vi "(SubVI)Waveform Editor_Import Manager.vi"(5 "New?":bool, 7 "Sampling Rate In":dbl, 8 "error in (no error)":errorcluster caption="에러 입력(에러 없음)", 10 "File Path":path, 11 "WAV File.lvclass":refnum<class "WAV File.lvclass">) -> (0 "error out":errorcluster caption="에러 출력", 2 "Apply?":bool, 3 "*.WAV Data":refnum<class "WAV File.lvclass">)   [LabVIEW 2020]
uses:
  Libraries/Waveform Obj Class/WAV File/WAV File.lvclass
  <vilib>/Utility/miscctls.llb/LVPointTypeDef.ctl
  Libraries/Waveform Obj Class/WAV File/WAV File.lvclass/WAV File.ctl
  Libraries/Waveform Obj Class/Waveform File/Waveform File.lvclass/Waveform File.ctl
  Libraries/Waveform Obj Class/Waveform Obj/Waveform Obj.lvclass/Waveform Obj.ctl
  Libraries/Waveform Obj Class/WAV File/Accessors/Read sound format.vi
  Libraries/Waveform Obj Class/Waveform File/Accessors/Read channel.vi
  Libraries/Waveform Obj Class/Waveform Obj/Accessors/Read voltage range.vi
  Libraries/Waveform Obj Class/Waveform Obj/Accessors/Read wait.vi
  Libraries/Waveform Obj Class/Waveform Obj/Accessors/Write sampling rate.vi
  Libraries/Waveform Obj Class/Waveform File/Accessors/Write channel.vi
  Libraries/Waveform Obj Class/WAV File/Accessors/Write normalize.vi
  Libraries/Waveform Obj Class/Waveform Obj/Accessors/Write wait.vi
  Libraries/Waveform Obj Class/Waveform Obj/Accessors/Write voltage range.vi
  Variables/(Var)System Variables.vi
  Libraries/Haptic IC Class/Haptic IC/Haptic IC.lvclass
panel:
  in  "Wait":u8(ring) items=["0us", "166us", "332us", "498us", "664us", "830us", "996us", "1162us", "1328us", "1494us", "1660us", "1826us", "1992us", "2158us", "2324us", "2490us"]
  in  "Normalize":bool=TRUE
  out "Bits per Sample":i32 caption="Bits / Sample"
  in  "Apply":bool
  out "Sampling Rate":dbl format="%#pHz"
  out "Graph":waveform(dbl)[](graph)
  in  "Voltage Range":dbl(ring) caption="VD Clamp" items=["0.00V"=0.0, "0.04V"=0.04, "0.08V"=0.08, "0.12V"=0.12, "0.16V"=0.16, "0.20V"=0.2, "0.24V"=0.24, "0.28V"=0.28, "0.32V"=0.32, "0.36V"=0.36, "0.40V"=0.4, "0.44V"=0.44, "0.48V"=0.48, "0.52V"=0.52, "0.56V"=0.56, "0.60V"=0.6, "0.64V"=0.64, "0.68V"=0.68, "0.72V"=0.72, "0.76V"=0.76, "0.80V"=0.8, "0.84V"=0.84, "0.88V"=0.88, "0.92V"=0.92, "0.96V"=0.96, "1.00V"=1.0, "1.04V"=1.04, "1.08V"=1.08, "1.12V"=1.12, "1.16V"=1.16, "1.20V"=1.2, "1.24V"=1.24, "1.28V"=1.28, "1.32V"=1.32, "1.36V"=1.36, "1.40V"=1.4, "1.44V"=1.44, "1.48V"=1.48, "1.52V"=1.52, "1.56V"=1.56, "1.60V"=1.6, "1.64V"=1.64, "1.68V"=1.68, "1.72V"=1.72, "1.76V"=1.76, "1.80V"=1.8, "1.84V"=1.84, "1.88V"=1.88, "1.92V"=1.92, "1.96V"=1.96, "2.00V"=2.0, "2.04V"=2.04, "2.08V"=2.08, "2.12V"=2.12, "2.16V"=2.16, "2.20V"=2.2, "2.24V"=2.24, "2.28V"=2.28, "2.32V"=2.32, "2.36V"=2.36, "2.40V"=2.4, "2.44V"=2.44, "2.48V"=2.48, "2.52V"=2.52, "2.56V"=2.56, "2.60V"=2.6, "2.64V"=2.64, "2.68V"=2.68, "2.72V"=2.72, "2.76V"=2.76, "2.80V"=2.8, "2.84V"=2.84, "2.88V"=2.88, "2.92V"=2.92, "2.96V"=2.96, "3.00V"=3.0, "3.04V"=3.04, "3.08V"=3.08, "3.12V"=3.12, "3.16V"=3.16, "3.20V"=3.2, "3.24V"=3.24, "3.28V"=3.28, "3.32V"=3.32, "3.36V"=3.36, "3.40V"=3.4, "3.44V"=3.44, "3.48V"=3.48, "3.52V"=3.52, "3.56V"=3.56, "3.60V"=3.6, "3.64V"=3.64, "3.68V"=3.68, "3.72V"=3.72, "3.76V"=3.76, "3.80V"=3.8, "3.84V"=3.84, "3.88V"=3.88, "3.92V"=3.92, "3.96V"=3.96, "4.00V"=4.0, "4.04V"=4.04, "4.08V"=4.08, "4.12V"=4.12, "4.16V"=4.16, "4.20V"=4.2, "4.24V"=4.24, "4.28V"=4.28, "4.32V"=4.32, "4.36V"=4.36, "4.40V"=4.4, "4.44V"=4.44, "4.48V"=4.48, "4.52V"=4.52, "4.56V"=4.56, "4.60V"=4.6, "4.64V"=4.64, "4.68V"=4.68, "4.72V"=4.72, "4.76V"=4.76, "4.80V"=4.8, "4.84V"=4.84, "4.88V"=4.88, "4.92V"=4.92, "4.96V"=4.96, "5.00V"=5.0, "5.04V"=5.04, "5.08V"=5.08, "5.12V"=5.12, "5.16V"=5.16, "5.20V"=5.2, "5.24V"=5.24, "5.28V"=5.28, "5.32V"=5.32, "5.36V"=5.36, "5.40V"=5.4, "5.44V"=5.44, "5.48V"=5.48, "5.52V"=5.52, "5.56V"=5.56, "5.60V"=5.6, "5.64V"=5.64, "5.68V"=5.68, "5.72V"=5.72, "5.76V"=5.76, "5.80V"=5.8, "5.84V"=5.84, "5.88V"=5.88, "5.92V"=5.92, "5.96V"=5.96, "6.00V"=6.0, "6.04V"=6.04, "6.08V"=6.08, "6.12V"=6.12, "6.16V"=6.16, "6.20V"=6.2, "6.24V"=6.24, "6.28V"=6.28, "6.32V"=6.32, "6.36V"=6.36, "6.40V"=6.4, "6.44V"=6.44, "6.48V"=6.48, "6.52V"=6.52, "6.56V"=6.56, "6.60V"=6.6, "6.64V"=6.64, "6.68V"=6.68, "6.72V"=6.72, "6.76V"=6.76, "6.80V"=6.8, "6.84V"=6.84, "6.88V"=6.88, "6.92V"=6.92, "6.96V"=6.96, "7.00V"=7.0, "7.04V"=7.04, "7.08V"=7.08, "7.12V"=7.12, "7.16V"=7.16, "7.20V"=7.2, "7.24V"=7.24, "7.28V"=7.28, "7.32V"=7.32, "7.36V"=7.36, "7.40V"=7.4, "7.44V"=7.44, "7.48V"=7.48, "7.52V"=7.52, "7.56V"=7.56, "7.60V"=7.6, "7.64V"=7.64, "7.68V"=7.68, "7.72V"=7.72, "7.76V"=7.76, "7.80V"=7.8, "7.84V"=7.84, "7.88V"=7.88, "7.92V"=7.92, "7.96V"=7.96, "8.00V"=8.0, "8.04V"=8.04, "8.08V"=8.08, "8.12V"=8.12, "8.16V"=8.16, "8.20V"=8.2, "8.24V"=8.24, "8.28V"=8.28, "8.32V"=8.32, "8.36V"=8.36, "8.40V"=8.4, "8.44V"=8.44, "8.48V"=8.48, "8.52V"=8.52, "8.56V"=8.56, "8.60V"=8.6, "8.64V"=8.64, "8.68V"=8.68, "8.72V"=8.72, "8.76V"=8.76, "8.80V"=8.8, "8.84V"=8.84, "8.88V"=8.88, "8.92V"=8.92, "8.96V"=8.96, "9.00V"=9.0, "9.04V"=9.04, "9.08V"=9.08, "9.12V"=9.12, "9.16V"=9.16, "9.20V"=9.2, "9.24V"=9.24, "9.28V"=9.28, "9.32V"=9.32, "9.36V"=9.36, "9.40V"=9.4, "9.44V"=9.44, "9.48V"=9.48, "9.52V"=9.52, "9.56V"=9.56, "9.60V"=9.6, "9.64V"=9.64, "9.68V"=9.68, "9.72V"=9.72, "9.76V"=9.76, "9.80V"=9.8, "9.84V"=9.84, "9.88V"=9.88, "9.92V"=9.92, "9.96V"=9.96, "10.00V"=10.0, "10.04V"=10.04, "10.08V"=10.08, "10.12V"=10.12, "10.16V"=10.16, "10.20V"=10.2]
  out "Freq":dbl caption="Sampling Rate" format="%#pHz"
  in  "Channel":i32(ring) items=["0"]
  # "Import Manager"
  # "File Info"
  # "Resampling"
  # "Setting"
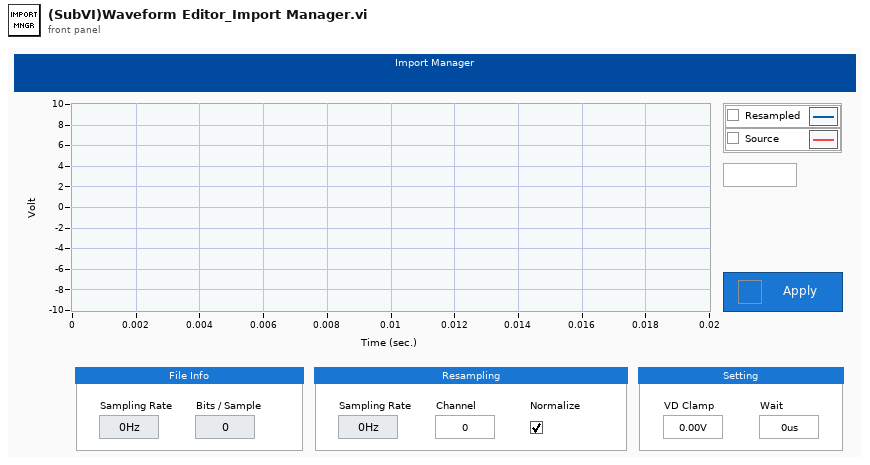
[diagram p1: front panel]
types:
  T1 = typedef "LVPointTypeDef.ctl" = cluster{"Horizontal":i16, "Vertical":i16}
  T2 = typedef "LVStringsAndValuesArrayTypeDef_DBL.ctl" = cluster{"String":string, "Value":dbl}[]
  T3 = typedef "LVStringsAndValuesArrayTypeDef_U8.ctl" = cluster{"String":string, "Value":u8}[]
  T4 = typedef "Sound Data Format.ctl" = cluster{"sample rate (S/s)":dbl, "number of channels":i32, "bits per sample":i32}
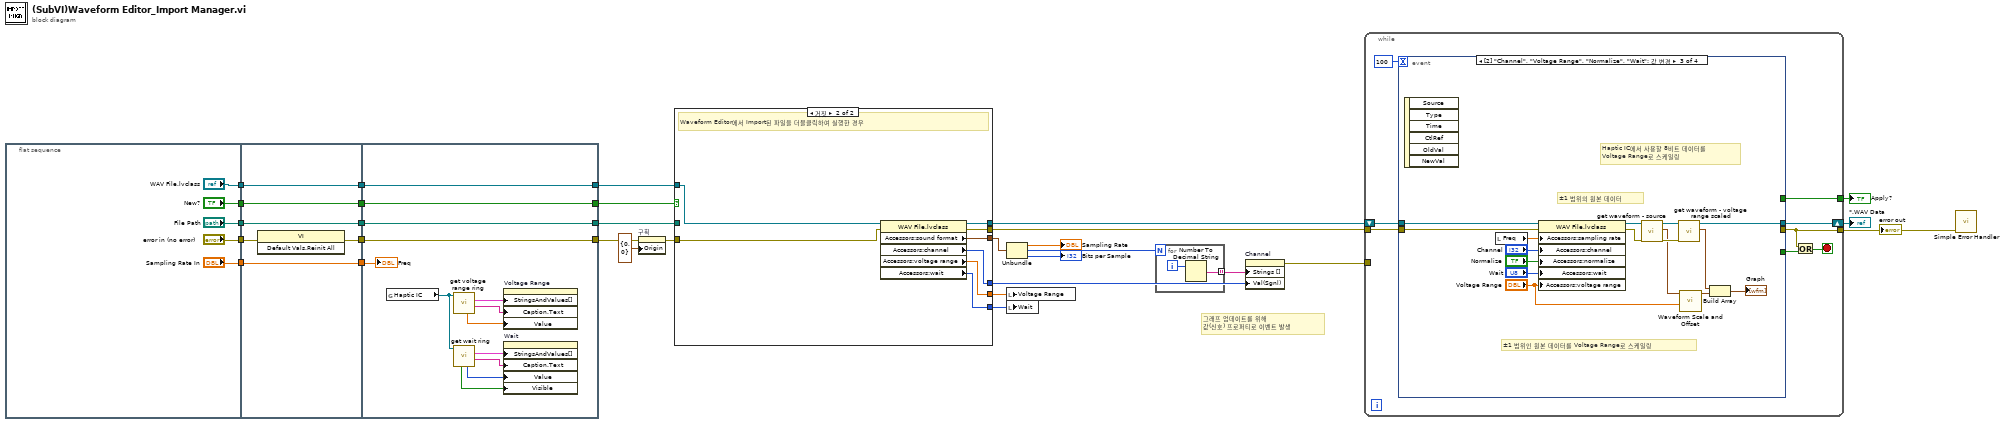
[diagram p0: block diagram]
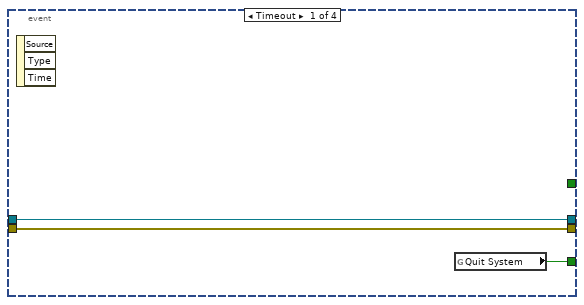
[diagram p2: hidden frame]
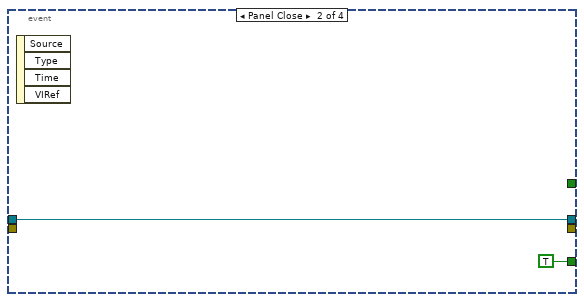
[diagram p3: hidden frame]
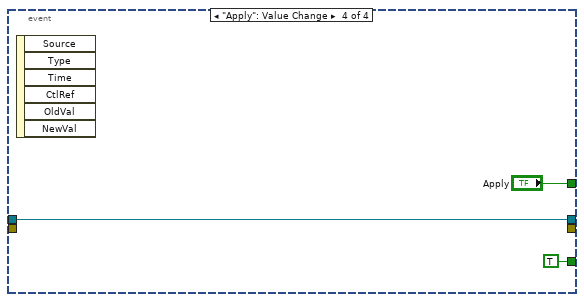
[diagram p4: hidden frame]
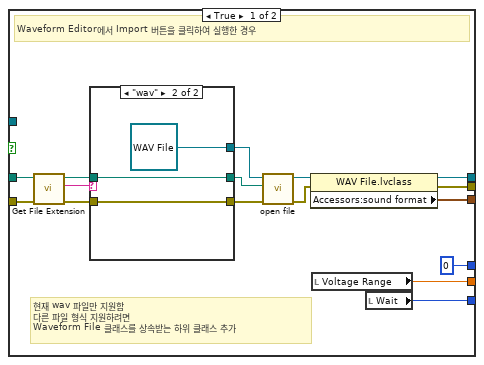
[diagram p5: hidden frame]
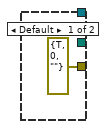
[diagram p6: hidden frame]
diagram:
  # "그래프 업데이트를 위해\n값(신호) 프로퍼티로 이벤트 발생"
  n1 = flat-sequence {
    tunnel: ["error in (no error)"] -> w26
    tunnel: ["File Path"] -> w25
    tunnel: ["Sampling Rate In"] -> w20
    tunnel: ["New?"] -> w14
    tunnel: ["WAV File.lvclass"] -> w12
    tunnel: w26 -> [w40]
    tunnel: w25 -> [w39]
    tunnel: [w41] -> w23
    tunnel: [w39] -> w22
    tunnel: [w38] -> w21
    tunnel: w20 -> [w38]
    tunnel: [w37] -> w15
    tunnel: w14 -> [w37]
    tunnel: [w36] -> w13
    tunnel: w12 -> [w36]
    tunnel: [w53] -> w24
    tunnel: [w54] -> w30
    tunnel: w23 -> [w54]
    tunnel: w22 -> [w53]
    tunnel: w21 -> [w52]
    tunnel: [w51] -> w11
    tunnel: w15 -> [w51]
    tunnel: [w50] -> w10
    tunnel: w13 -> [w50]
    frame #0 {
    }
    frame #1 {
      n2 = invoke class="VI" method="Default Vals.Reinit All"(error in=w40) -> (error out=w41:errorcluster)  [unwired: 2 in, 2 out]
    }
    frame #2 {
      n3 = global read "(Var)System Variables.vi" "Haptic IC"() -> (w48:refnum<class "Haptic IC.lvclass">)
      n4 = call-dynamic "get voltage range ring.vi"("Haptic IC 입력"=w48) -> ("caption"=w43:string, "strings & values"=w42:T2, "read value"=w49:dbl)  [unwired: 6 in, 2 out]
      n5 = call-dynamic "get wait ring.vi"("Haptic IC 입력"=w48) -> ("caption"=w46:string, "strings & values"=w47:T3, "default value"=w45:u8, "using"=w44:bool)  [unwired: 5 in, 2 out]
      n6 = property on="Voltage Range" class="Ring (엄격한)"("StringsAndValues[]"=w42, "Caption.Text"=w43, "Value"=w49) -> ()  [unwired: 2 in, 2 out]
      n7 = property on="Wait" class="Ring (엄격한)"("StringsAndValues[]"=w47, "Caption.Text"=w46, "Value"=w45, "Visible"=w44) -> ()  [unwired: 2 in, 2 out]
      "Freq" <- w52
    }
  }
  n8 = property on="구획" class="Pane"(error in=w30, "Origin"=T1 {"Horizontal"=0, "Vertical"=0} ("원점")) -> (error out=w19:errorcluster)  [unwired: 1 in, 1 out]
  n9 = case shown="거짓" w11 {
    tunnel: [w65 w82] -> w29
    tunnel: [w63 w81] -> w28
    tunnel: [w62 w80] -> w8
    tunnel: w24 -> [w61 _]
    tunnel: w19 -> [w60 w79]
    tunnel: w10 -> [_ w78]
    tunnel: [0 ("값(신호)") w77] -> w5
    tunnel: [w55 w76] -> w2
    tunnel: [w56 w75] -> w1
    frame True {
      # "현재 wav 파일만 지원함\n다른 파일 형식 지원하려면 \nWaveform File 클래스를 상속받는 하위 클래스 추가"
      # "Waveform Editor에서 Import 버튼을 클릭하여 실행한 경우"
      n10 = call <vilib>:"Get File Extension.vi"("error in (no error)"=w60, "file"=w61) -> ("error out"=w70:errorcluster, "lowercase file extension"=w69:string, "dup file"=w67:path)  [unwired: 5 in, 2 out]
      n11 = case shown="\"wav\"" w69 {
        tunnel: w70 -> [_ w74]
        tunnel: [errorcluster {"status"=TRUE, "code"=0, "source"=""} ("error out") w74] -> w68
        tunnel: [_ refnum<class "WAV File.lvclass"> refnum ("WAV File.lvclass")] -> w66
        tunnel: w67 -> [_ w72]
        tunnel: [_ w72] -> w59
        frame Default {
        }
        frame "wav" {
        }
      }
      n12 = call-dynamic "open file.vi"("error in (no error)"=w68, "file path"=w59, "WAV File 입력"=w66) -> ("error out"=w58:errorcluster, "WAV File 출력"=w64:refnum<class "WAV File.lvclass">)  [unwired: 7 in]
      n13 = property class="WAV File.lvclass"(reference=w64, error in=w58) -> (reference out=w63:refnum<class "WAV File.lvclass">, error out=w65:errorcluster, "Accessors:sound format"=w62:T4)
      n14 = local read "Voltage Range"() -> (w55:dbl)
      n15 = local read "Wait"() -> (w56:u8)
    }
    frame False {
      # "Waveform Editor에서 Import된 파일을 더블클릭하여 실행한 경우"
      n16 = property class="WAV File.lvclass"(reference=w78, error in=w79) -> (reference out=w81:refnum<class "WAV File.lvclass">, error out=w82:errorcluster, "Accessors:sound format"=w80:T4, "Accessors:channel"=w77:i32, "Accessors:voltage range"=w76:dbl, "Accessors:wait"=w75:u8)
    }
  }
  n17 = Unbundle(w8) -> ("sample rate (S/s)"=→"Sampling Rate":dbl, "number of channels"=w6:i32, "bits per sample"=→"Bits per Sample":i32)
  n18 = local write "Voltage Range"(w2) -> ()
  n19 = local write "Wait"(w1) -> ()
  n20 = for {
    N: w6 -> [_]
    tunnel: [w83] -> w27 mode=indexing
    i -> [w84]
    n21 = Number To Decimal String(number=w84) -> (decimal integer string=w83:string)  [unwired: 1 in]
  }
  n22 = property on="Channel" class="Ring (엄격한)"("Strings []"=w27, "Val(Sgnl)"=w5) -> (error out=w3:errorcluster)  [unwired: 2 in, 1 out]
  n23 = while {
    tunnel: w29 -> [w89]
    tunnel: [w86] -> w9
    shift-right: [w91] -> w16
    shift-left: w28 -> [w90]
    tunnel: [w85] -> w17
    tunnel: w3 -> [_]
    stop <- w87 stop-if-true
    n24 = event shown="[2] \"Channel\", \"Voltage Range\", \"Normalize\", \"Wait\": 값 변경" {
      selector: _ -> [_ _ _ _]
      dyn-events: _ -> [_ _ _ _]
      timeout: 100 -> [_ _ _ _]
      tunnel: [w95 w97 w105 w116] -> w91
      tunnel: w90 -> [w95 w97 w113 w116]
      tunnel: w89 -> [w94 _ w108 _]
      tunnel: [w94 _ _ _] -> w86
      tunnel: [w93 TRUE _ TRUE] -> w88
      tunnel: [_ _ _ "Apply"] -> w85
      event Timeout {
        n25 = event-data() -> ()  [unwired: 1 in, 3 out]
        n26 = global read "(Var)System Variables.vi" "Quit System"() -> (w93:bool)
      }
      event Panel Close {
        n27 = event-data() -> ()  [unwired: 1 in, 4 out]
      }
      event "Channel", "Voltage Range", "Normalize", "Wait": Value Change {
        # "±1 범위의 원본 데이터"
        # "Haptic IC에서 사용할 8비트 데이터를\nVoltage Range로 스케일링"
        # "±1 범위인 원본 데이터를 Voltage Range로 스케일링"
        n28 = event-data() -> ()  [unwired: 1 in, 6 out]
        n29 = local read "Freq"() -> (w107:dbl)
        n30 = property class="WAV File.lvclass"(reference=w113, error in=w108, "Accessors:sampling rate"=w107, "Accessors:channel"="Channel", "Accessors:normalize"="Normalize", "Accessors:wait"="Wait", "Accessors:voltage range"="Voltage Range") -> (reference out=w112:refnum<class "WAV File.lvclass">, error out=w109:errorcluster)
        n31 = call-dynamic "get waveform - source.vi"("error in (no error)"=w109, "WAV File 입력"=w112) -> ("error out"=w104:errorcluster, "waveform"=w102:waveform(dbl), "WAV File 출력"=w110:refnum<class "WAV File.lvclass">)  [unwired: 7 in]
        n32 = call-dynamic "get waveform - voltage range scaled.vi"("error in (no error)"=w104, "WAV File 입력"=w110) -> ("scaled waveform"=w103:waveform(dbl), "WAV File 출력"=w105:refnum<class "WAV File.lvclass">)  [unwired: 7 in, 1 out]
        n33 = call <vilib>:"Waveform Scale and Offset.vi"("scale"="Voltage Range", "waveform in"=w102) -> ("waveform out"=w100:waveform(dbl))  [unwired: 8 in, 1 out]
        n34 = Build Array(w103, w100) -> (→"Graph":waveform(dbl)[])
      }
      event "Apply": Value Change {
        n35 = event-data() -> ()  [unwired: 1 in, 6 out]
      }
    }
    n36 = Or(x=w86, y=w88) -> (x .or. y?=w87:bool)
  }
  "error out" <- w9
  "Apply?" <- w17
  "*.WAV Data" <- w16
  n37 = call <vilib>:"Simple Error Handler.vi"("error in (no error)"=w9) -> ()  [unwired: 4 in, 5 out]
